vi "gate_controller.vi"(10 "Numerical Argument":dbl, 11 "Command":T1(ring)=enum."Read Voltage") -> (3 "Response":string)   [LabVIEW 2021]
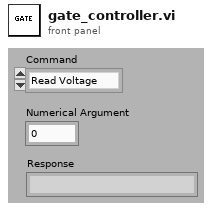
[diagram p1: front panel]
types:
  T1 = enum16{"Set Voltage", "Read Voltage", "Read Setpoint", "Read Current", "Output On", "Output Off"}
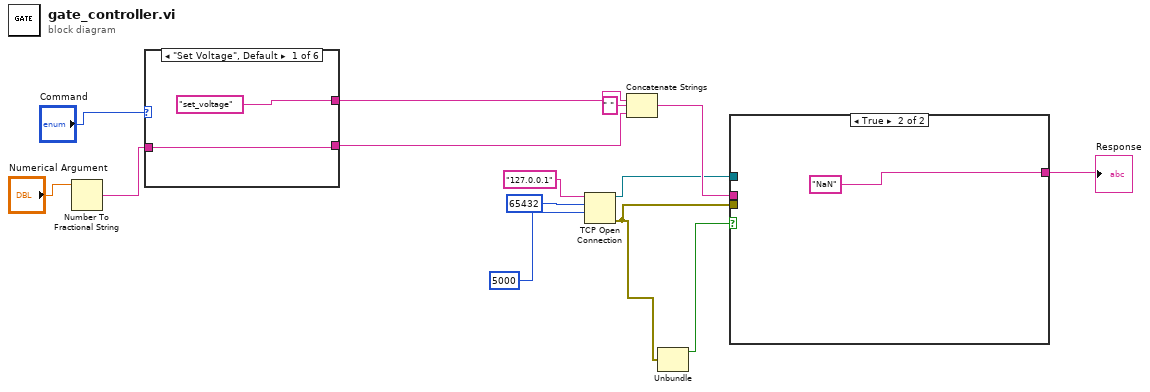
[diagram p0: block diagram]
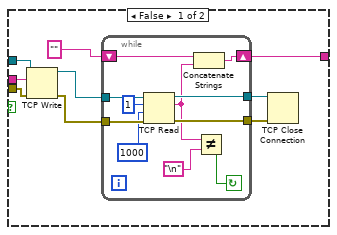
[diagram p2: hidden frame]
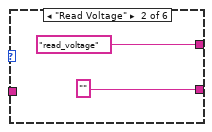
[diagram p3: hidden frame]
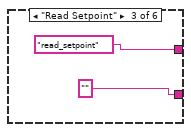
[diagram p4: hidden frame]
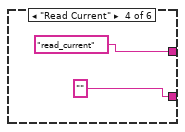
[diagram p5: hidden frame]
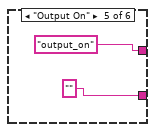
[diagram p6: hidden frame]
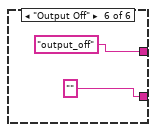
[diagram p7: hidden frame]
diagram:
  n1 = Number To Fractional String(number="Numerical Argument") -> (F-format string=w8:string)  [unwired: 3 in]
  n2 = case shown="\"Set Voltage\", Default" "Command" {
    tunnel: ["set_voltage" ("data in") "read_voltage" ("data in") "read_setpoint" ("data in") "read_current" ("data in") "output_on" ("data in") "output_off" ("data in")] -> w12
    tunnel: [w15 "" ("string") "" ("string") "" ("string") "" ("string") "" ("string")] -> w9
    tunnel: w8 -> [w15 _ _ _ _ _]
    frame "Set Voltage", Default {
    }
    frame "Read Voltage" {
    }
    frame "Read Setpoint" {
    }
    frame "Read Current" {
    }
    frame "Output On" {
    }
    frame "Output Off" {
    }
  }
  n3 = TCP Open Connection(address="127.0.0.1", remote port or service name=u16 65432, timeout ms (60000)=5000) -> (connection ID=w1:refnum<k5>, error out=w3:errorcluster)  [unwired: 2 in]
  n4 = Concatenate Strings(w12, " " ("string"), w9) -> (w2:string)
  n5 = Unbundle(w3) -> ("status"=w4:bool)  [unwired: 2 out]
  n6 = case shown="True" w4 {
    tunnel: [w32 "NaN"] -> w5
    tunnel: w3 -> [w31 _]
    tunnel: w2 -> [w30 _]
    tunnel: w1 -> [w29 _]
    frame False {
      n7 = TCP Write(connection ID=w29, data in=w30, error in (no error)=w31) -> (connection ID out=w27:refnum<k5>, error out=w28:errorcluster)  [unwired: 1 in, 1 out]
      n8 = while {
        tunnel: w28 -> [w46]
        tunnel: w27 -> [w45]
        tunnel: [w44] -> w35
        tunnel: [w43] -> w34
        shift-right: [w39] -> w32
        shift-left: "" ("string") -> [w40]
        stop <- w38 continue-if-true
        n9 = TCP Read(connection ID=w45, bytes to read=1, error in (no error)=w46, 9:1000 ("timeout ms (25000)")) -> (connection ID out=w43:refnum<k5>, data out=w37:string, error out=w44:errorcluster)  [unwired: 1 in]
        n10 = Concatenate Strings(w40, w37) -> (w39:string)
        n11 = Not Equal?(x=w37, y="\n") -> (x != y?=w38:bool)
      }
      n12 = TCP Close Connection(connection ID=w34, error in (no error)=w35) -> ()  [unwired: 1 in, 2 out]
    }
    frame True {
    }
  }
  "Response" <- w5
